vi "GFITS_LibsimpleDataWrite.vi"(4 "bufptr":u64, 5 "nrows":i32, 6 "dtype":i32, 7 "ncols":i32, 8 "error in (no error)":errorcluster, 9 "ntries":i32=1, 11 "name":string) -> (0 "error out":errorcluster, 3 "ref out":u64)   [LabVIEW 2016]
uses:
  c/lib/libgfits.so
panel:
  in  "err":i32
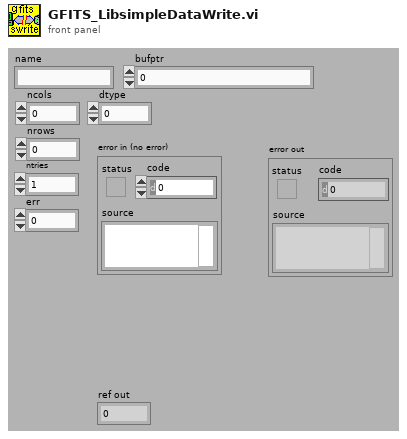
[diagram p1: front panel]
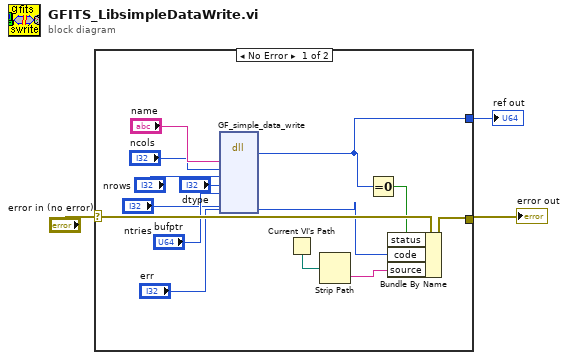
[diagram p0: block diagram]
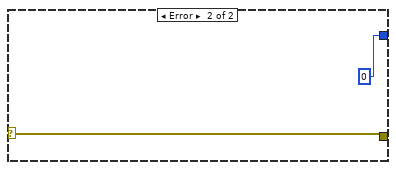
[diagram p2: hidden frame]
diagram:
  n1 = case shown="No Error" "error in (no error)" {
    selector: "error in (no error)" -> [w17 w19]
    tunnel: [w13 w19] -> w2
    tunnel: [w7 0] -> w1
    frame No Error {
      n2 = dll-call lib="home/simager/panview/PAN/Modules/GFITS/private/c/lib/libgfits.so" fn="GF_simple_data_write"("name"="name", "ncols"="ncols", "nrows"="nrows", "dtype"="dtype", "bufptr"="bufptr", "ntries"="ntries", "err"="err") -> ("return type"=w7:u64, "err"=w4:i32)  [unwired: 9 in, 2 out]
      n3 = Current VI's Path() -> (path=w15:path)
      n4 = Strip Path(path=w15) -> (name=w14:string)  [unwired: 1 out]
      n5 = Equal To 0?(x=w7) -> (x = 0?=w16:bool)
      n6 = Bundle By Name(cluster=w17, "status"=w16, "code"=w4, "source"=w14) -> (w13:errorcluster)
    }
    frame Error {
    }
  }
  "error out" <- w2
  "ref out" <- w1
